vi "AC Couple (1 Ch SGL WFM).vi"(8 "error in (no error)":errorcluster, 11 "Signal":waveform(sgl)) -> (0 "error out":errorcluster, 1 "DC":sgl, 3 "AC Coupled":waveform(sgl))   [LabVIEW 2017, in "VibrationAnalysisFunctions.lvlib"]
uses:
  <vilib>/addons/InsightCM/Utilities/Analysis/Vibration/VibrationAnalysisFunctions.lvlib
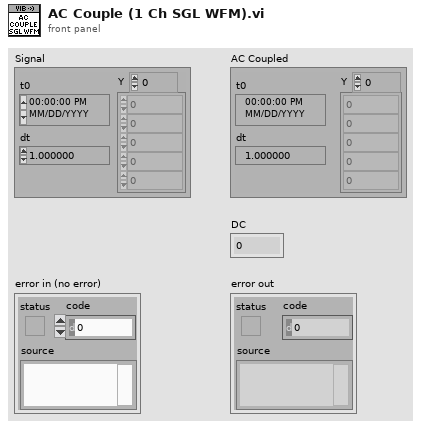
[diagram p1: front panel]
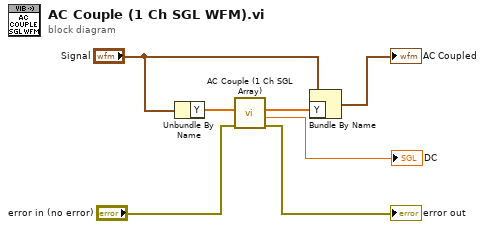
[diagram p0: block diagram]
diagram:
  n1 = Unbundle By Name("Signal") -> ("Y"=w5:sgl[])
  n2 = call <vilib>:"AC Couple (1 Ch SGL Array).vi"("error in (no error)"="error in (no error)", "Signal"=w5) -> ("error out"=→"error out":errorcluster, "DC"=→"DC":sgl, "AC Coupled"=w4:sgl[])  [unwired: 7 in]
  n3 = Bundle By Name(cluster="Signal", "Y"=w4) -> (→"AC Coupled":waveform(sgl))
